vi "node information.vi"(8 "error in":errorcluster, 11 "refnum in":T1) -> (0 "error out":errorcluster, 1 "global dvr ref":refnum<data-value>, 2 "my subscriptions[]":string[](array[string]), 3 "refnum in":T1, 4 "this node name":string, 5 "all active nodes[]":string[](array[string]))   [LabVIEW 2020, in "Publisher Subscriber.lvlib"]
uses:
  Publisher Subscriber.lvlib
  Controls/node refnum.ctl
  Controls/node dvr data.ctl
  Controls/data cluster.ctl
  Controls/subscription bank ref.ctl
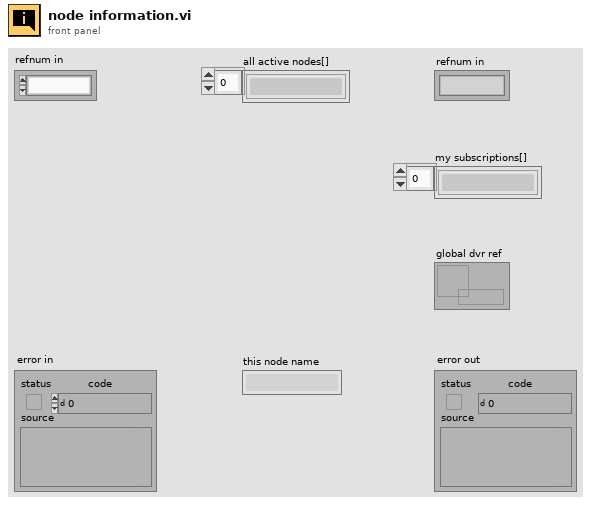
[diagram p1: front panel]
types:
  T1 = typedef "Publisher Subscriber.lvlib/node refnum.ctl" = refnum<k1>
  T2 = typedef "Publisher Subscriber.lvlib/node dvr data.ctl" = cluster{"queue ref":refnum<queue>, "Subscription Bank Ref":refnum<data-value>, "Command":string, "Data":variant, "Subscriptions []":set{string}, "Variables DVR Ref":refnum<data-value>}
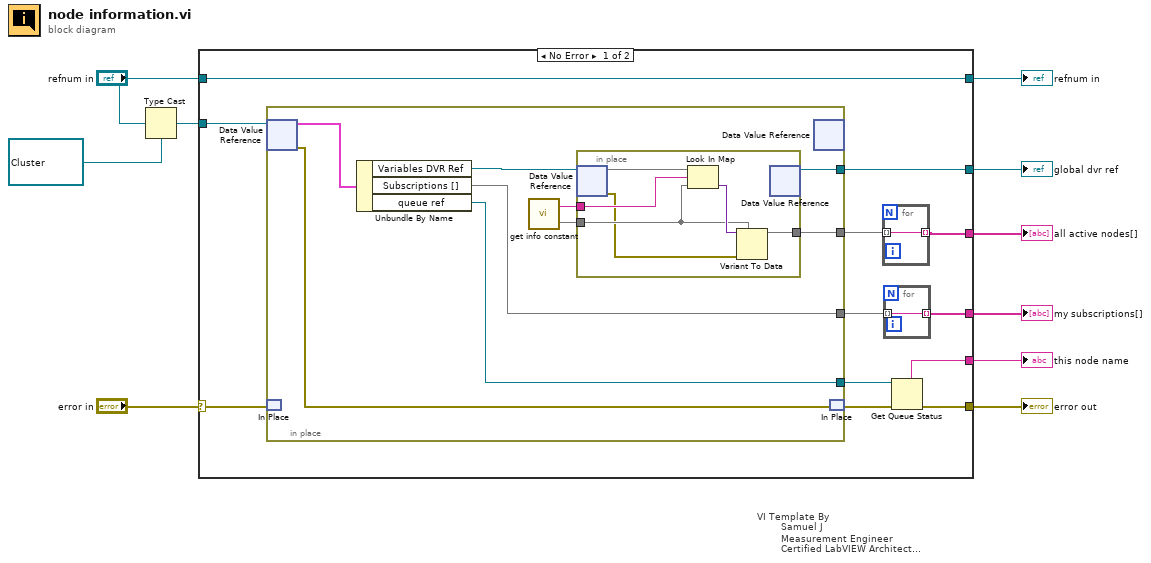
[diagram p0: block diagram]
diagram:
  n1 = Type Cast(type=refnum<data-value> refnum ("data value reference"), x="refnum in") -> (*(type *) &x=w7:refnum<data-value>)
  n2 = case "VI Template By\n        Samuel J\n        Measurement Engineer\n        Certified LabVIEW Architect\n        Vestas Technology R&D Chennai" shown="No Error" "error in" {
    selector: "error in" -> [w20 w41]
    tunnel: [w15 w41] -> w9
    tunnel: w7 -> [w21 _]
    tunnel: [w22 w40] -> w6
    tunnel: "refnum in" -> [w22 w40]
    tunnel: [w17 _] -> w4
    tunnel: [w19 _] -> w3
    tunnel: [w13 _] -> w2
    tunnel: [w11 _] -> w1
    frame No Error {
      n3 = in-place {
        in-place-border: [w24] -> w19
        in-place-border: [w30] -> w18
        in-place-border: [w28] -> w14
        in-place-border: [w23] -> w12
        n4 = in-place-dvr #1(w21) -> (w31:T2, w29:errorcluster)
        n5 = in-place-match #2(w20) -> ()  [unwired: 1 out]
        n6 = Unbundle By Name(w31) -> ("Variables DVR Ref"=w25:refnum<data-value>, "Subscriptions []"=w30:set{string}, "queue ref"=w28:refnum<queue>)
        n7 = call "get info constant.vi"() -> ("set"=w26:set{string}, "String"=w27:string)  [unwired: 4 in]
        n8 = in-place {
          in-place-border: w27 -> [w36]
          in-place-border: w26 -> [w34]
          in-place-border: [w32] -> w23
          n9 = in-place-dvr #3(w25) -> (w37:map{string, variant}, w33:errorcluster)
          n10 = Look In Map(map=w37, key=w36, default value=w34) -> (value=w35:variant)  [unwired: 1 out]
          n11 = Variant To Data(error in=w33, type=w34, Variant=w35) -> (data=w32:set{string})  [unwired: 1 out]
          n12 = in-place-dvr #3() -> (w24:refnum<data-value>)  [unwired: 1 in, 1 out]
        }
        n13 = in-place-dvr #1() -> ()  [unwired: 1 in, 2 out]
        n14 = in-place-match #2(w29) -> (w16:errorcluster)
      }
      n15 = for {
        tunnel: [w38] -> w11 mode=indexing
        tunnel: w12 -> [w38] mode=indexing
      }
      n16 = for {
        tunnel: [w39] -> w17 mode=indexing
        tunnel: w18 -> [w39] mode=indexing
      }
      n17 = Get Queue Status(queue=w14, error in (no error)=w16) -> (queue name=w13:string, error out=w15:errorcluster)  [unwired: 1 in, 6 out]
    }
    frame Error {
    }
  }
  "error out" <- w9
  "refnum in" <- w6
  "my subscriptions[]" <- w4
  "global dvr ref" <- w3
  "this node name" <- w2
  "all active nodes[]" <- w1
